vi "PH_IEEE1394Camera.set names of relevant attributes.vi"(1 "Bus Type":string) -> (0 "Relevant Cam Attributes":T1)   [LabVIEW 2014, in "PH_IEEE1394Camera.lvlib"]
uses:
  PH_IEEE1394Camera.lvlib
  PH_IEEE1394Camera.Relevant Cam Attributes.ctl
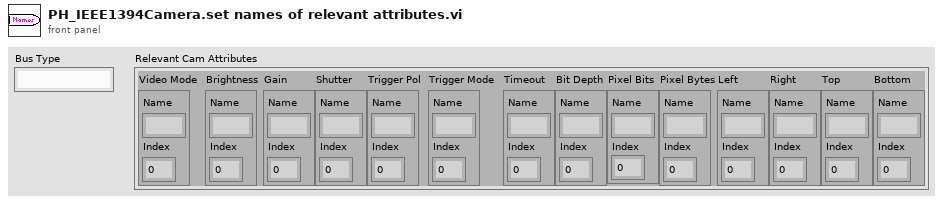
[diagram p1: front panel]
types:
  T1 = typedef "PH_IEEE1394Camera.lvlib/PH_IEEE1394Camera.Relevant Cam Attributes.ctl" = cluster{"Video Mode":cluster{"Name":string, "Index":i32}, "Brightness":cluster{"Name":string, "Index":i32}, "Gain":cluster{"Name":string, "Index":i32}, "Shutter":cluster{"Name":string, "Index":i32}, "Trigger Pol":cluster{"Name":string, "Index":i32}, "Trigger Mode":cluster{"Name":string, "Index":i32}, "Timeout":cluster{"Name":string, "Index":i32}, "Bit Depth":cluster{"Name":string, "Index":i32}, "Pixel Bits":cluster{"Name":string, "Index":i32}, "Pixel Bytes":cluster{"Name":string, "Index":i32}, "Left":cluster{"Name":string, "Index":i32}, "Right":cluster{"Name":string, "Index":i32}, "Top":cluster{"Name":string, "Index":i32}, "Bottom":cluster{"Name":string, "Index":i32}}
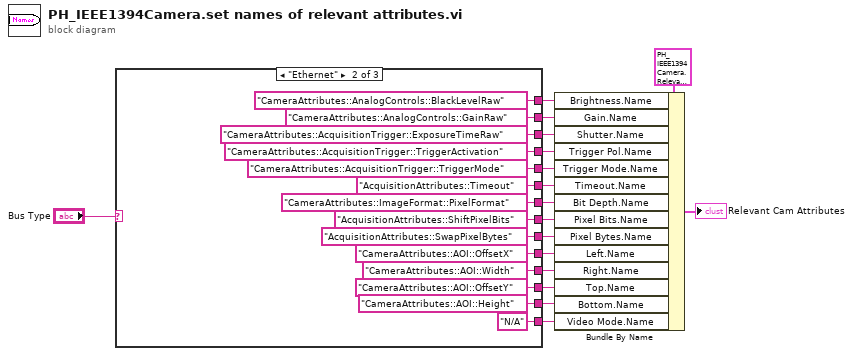
[diagram p0: block diagram]
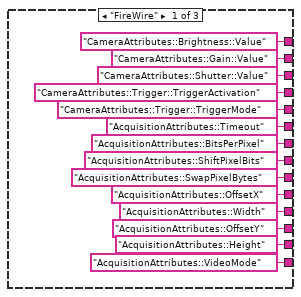
[diagram p2: hidden frame]
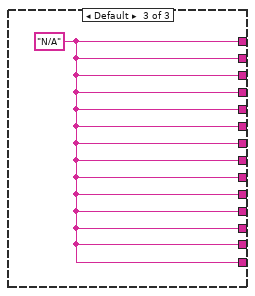
[diagram p3: hidden frame]
diagram:
  n1 = case shown="\"Ethernet\"" "Bus Type" {
    tunnel: ["AcquisitionAttributes::VideoMode" "N/A" w46] -> w14
    tunnel: ["CameraAttributes::Brightness::Value" "CameraAttributes::AnalogControls::BlackLevelRaw" w46] -> w13
    tunnel: ["CameraAttributes::Gain::Value" "CameraAttributes::AnalogControls::GainRaw" w46] -> w12
    tunnel: ["CameraAttributes::Shutter::Value" "CameraAttributes::AcquisitionTrigger::ExposureTimeRaw" w46] -> w11
    tunnel: ["CameraAttributes::Trigger::TriggerActivation" "CameraAttributes::AcquisitionTrigger::TriggerActivation" w46] -> w10
    tunnel: ["CameraAttributes::Trigger::TriggerMode" "CameraAttributes::AcquisitionTrigger::TriggerMode" w46] -> w9
    tunnel: ["AcquisitionAttributes::Timeout" "AcquisitionAttributes::Timeout" w46] -> w8
    tunnel: ["AcquisitionAttributes::BitsPerPixel" "CameraAttributes::ImageFormat::PixelFormat" w46] -> w7
    tunnel: ["AcquisitionAttributes::ShiftPixelBits" "AcquisitionAttributes::ShiftPixelBits" w46] -> w6
    tunnel: ["AcquisitionAttributes::SwapPixelBytes" "AcquisitionAttributes::SwapPixelBytes" w46] -> w5
    tunnel: ["AcquisitionAttributes::OffsetX" "CameraAttributes::AOI::OffsetX" w46] -> w4
    tunnel: ["AcquisitionAttributes::Width" "CameraAttributes::AOI::Width" w46] -> w3
    tunnel: ["AcquisitionAttributes::OffsetY" "CameraAttributes::AOI::OffsetY" w46] -> w2
    tunnel: ["AcquisitionAttributes::Height" "CameraAttributes::AOI::Height" w46] -> w1
    frame "FireWire" {
    }
    frame "Ethernet" {
    }
    frame Default {
      w46 = "N/A"
    }
  }
  n2 = Bundle By Name(cluster=T1 {"Video Mode"={"Name"="", "Index"=0}, "Brightness"={"Name"="", "Index"=0}, "Gain"={"Name"="", "Index"=0}, "Shutter"={"Name"="", "Index"=0}, "Trigger Pol"={"Name"="", "Index"=0}, "Trigger Mode"={"Name"="", "Index"=0}, "Timeout"={"Name"="", "Index"=0}, "Bit Depth"={"Name"="", "Index"=0}, "Pixel Bits"={"Name"="", "Index"=0}, "Pixel Bytes"={"Name"="", "Index"=0}, "Left"={"Name"="", "Index"=0}, "Right"={"Name"="", "Index"=0}, "Top"={"Name"="", "Index"=0}, "Bottom"={"Name"="", "Index"=0}} ("Relevant Cam Attributes"), "Brightness.Name"=w13, "Gain.Name"=w12, "Shutter.Name"=w11, "Trigger Pol.Name"=w10, "Trigger Mode.Name"=w9, "Timeout.Name"=w8, "Bit Depth.Name"=w7, "Pixel Bits.Name"=w6, "Pixel Bytes.Name"=w5, "Left.Name"=w4, "Right.Name"=w3, "Top.Name"=w2, "Bottom.Name"=w1, "Video Mode.Name"=w14) -> (→"Relevant Cam Attributes":T1)
